vi "Capture@LoadFile__Parameter.vi"(1 "ParamterIn":string) -> (0 "ParamterOut":string)   [LabVIEW 2020]
uses:
  MainFrame/Global.vi
panel:
  out "All Files in Dir":path[](array[path])
  out "Image":T1(plugin-control)
  in  "Picture":string(combo)
  in  "CamName":string(combo)
  in  "Confirm":bool
  # "Capture@General $Capture,$Picture"
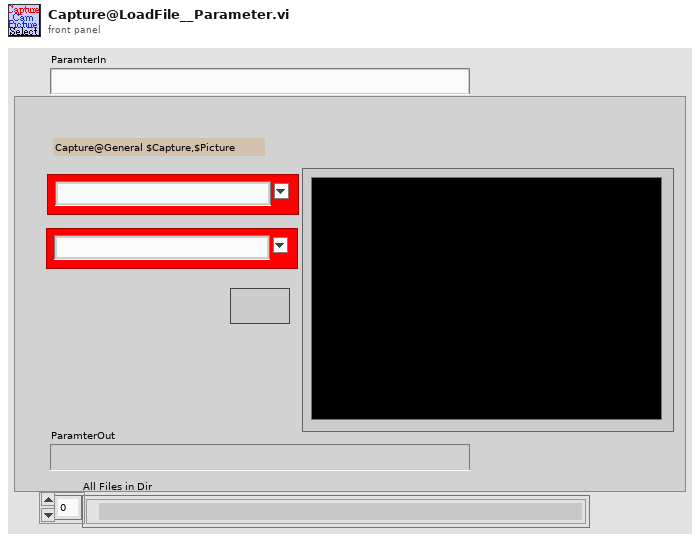
[diagram p1: front panel]
types:
  T1 = typedef "IMAQ Image.ctl" = refnum<image>
  T2 = typedef "Image Type" = u32
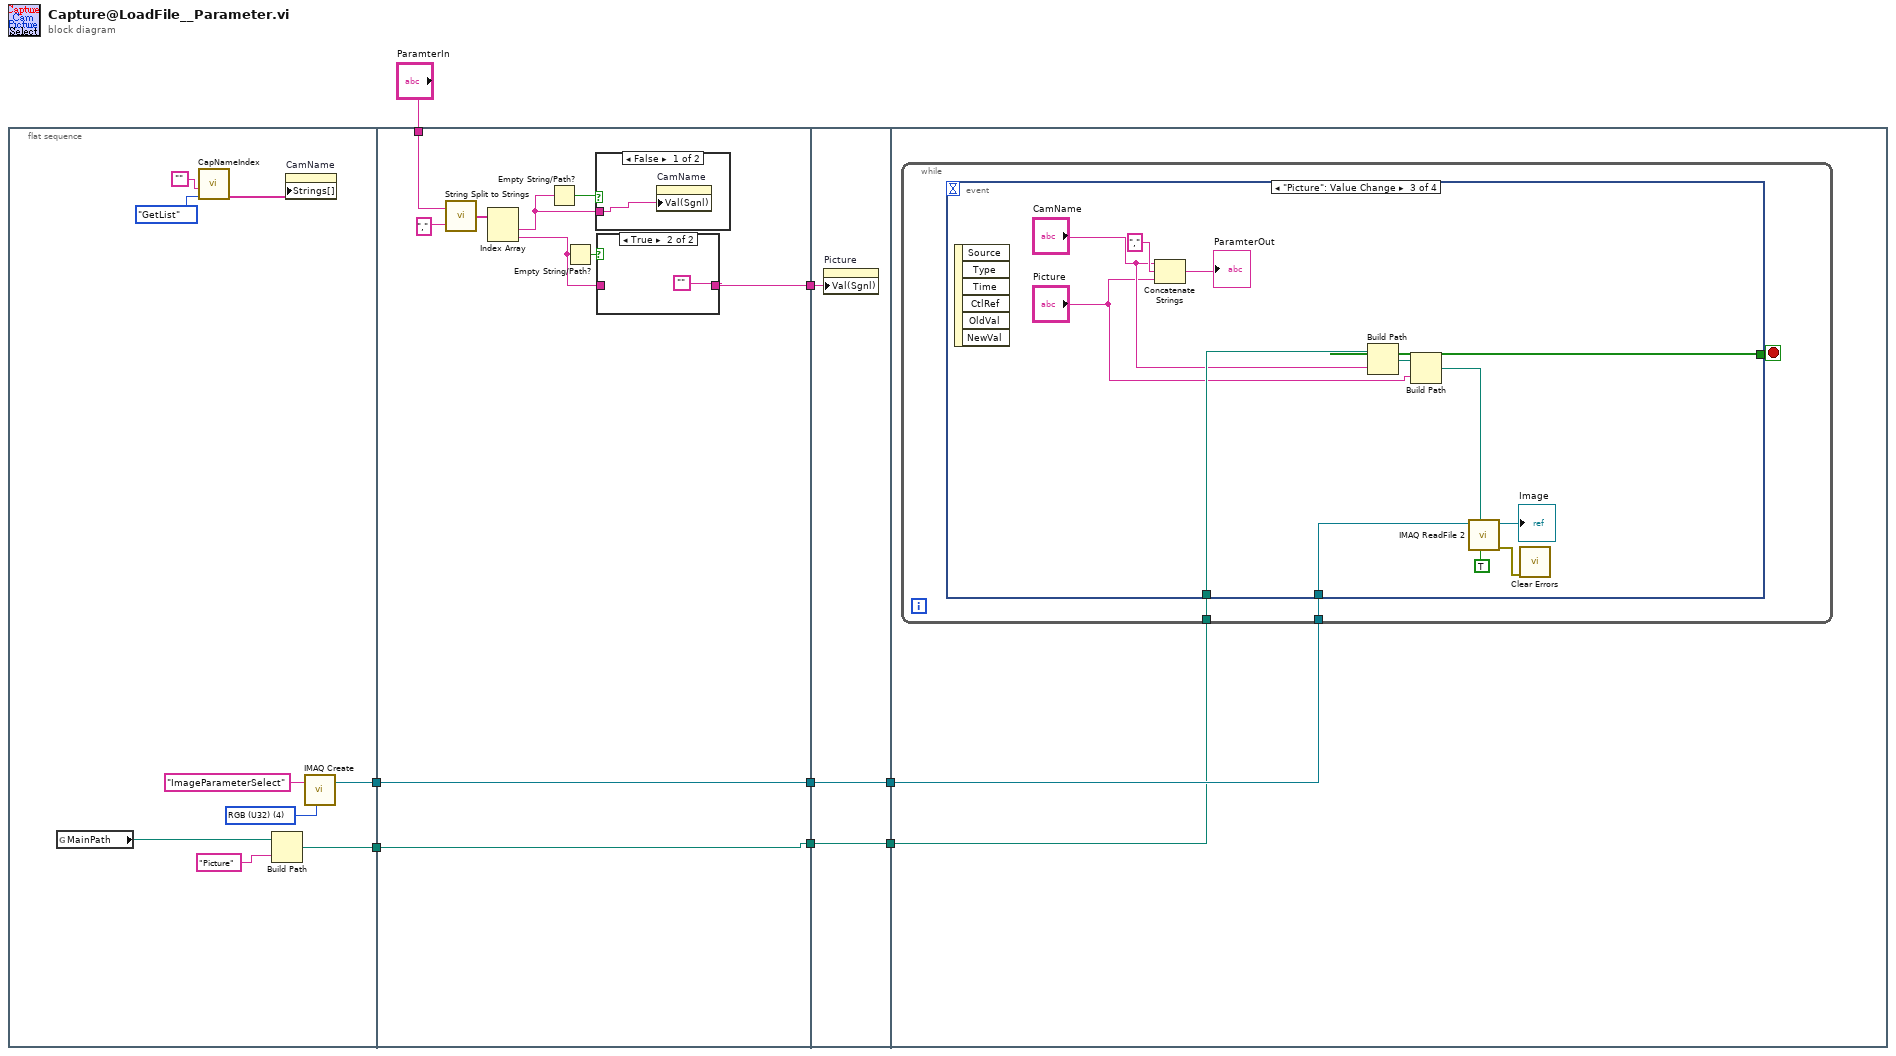
[diagram p0: block diagram]
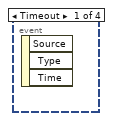
[diagram p4: hidden frame]
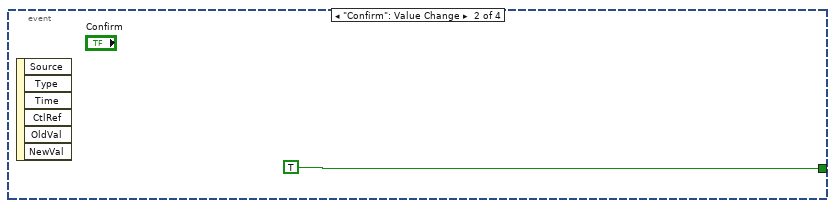
[diagram p5: hidden frame]
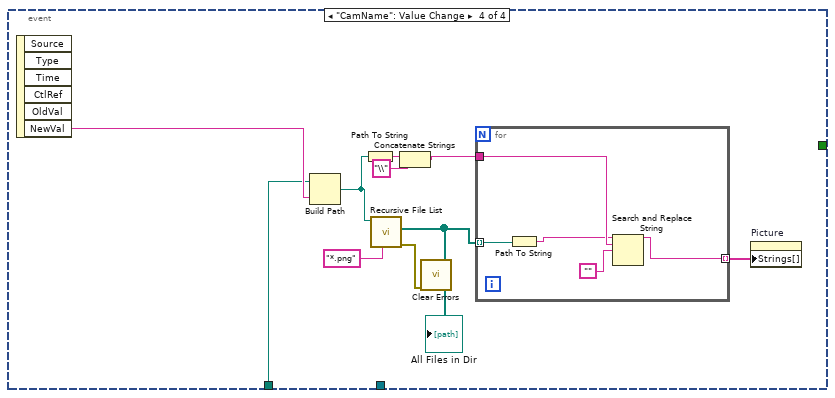
[diagram p6: hidden frame]
diagram:
  n1 = flat-sequence {
    tunnel: [w13] -> w7
    tunnel: [w11] -> w2
    tunnel: "ParamterIn" -> [w25]
    tunnel: w7 -> [w21]
    tunnel: [w21] -> w6
    tunnel: [w19] -> w3
    tunnel: w2 -> [w19]
    tunnel: [w18] -> w1
    tunnel: w6 -> [w33]
    tunnel: [w33] -> w5
    tunnel: [w32] -> w4
    tunnel: w3 -> [w32]
    tunnel: w1 -> [w31]
    tunnel: w5 -> [w35]
    tunnel: w4 -> [w34]
    frame #0 {
      w9 = T2 4 items=["Grayscale (U8)", "Grayscale (I16)", "Grayscale (SGL)", "Complex (CSG)", "RGB (U32)", "HSL (U32)", "RGB (U64)", "Grayscale (U16)"] ("Image Type")
      n2 = global read "Global.vi" "MainPath"() -> (w10:path)
      n3 = call "CapNameIndex.vi"("OP"=enum16{"AddCam", "GetIndex", "Init", "GetList"}."GetList", "CamName"="") -> ("DeviceList"=w16:string[])  [unwired: 2 in, 3 out]
      n4 = Build Path(base path=w10, name or relative path="Picture") -> (appended path=w11:path)
      n5 = property on="CamName" class="CmbBox"("Strings[]"=w16) -> ()  [unwired: 2 in, 2 out]
      n6 = call "IMAQ Create"("Image Name"="ImageParameterSelect", "Image Type"=w9) -> ("New Image"=w13:T1)  [unwired: 3 in, 1 out]
    }
    frame #1 {
      n7 = call "String Split to Strings.vi"("search string/char (-)"=",", "String"=w25) -> ("Array"=w27:string[])
      n8 = Index Array(array=w27) -> (element #1=w20:string, element #2=w22:string)  [unwired: 2 in]
      n9 = Empty String/Path?(string/path=w20) -> (empty?=w24:bool)
      n10 = Empty String/Path?(string/path=w22) -> (empty?=w23:bool)
      n11 = case shown="False" w24 {
        tunnel: w20 -> [w30 _]
        frame False {
          n12 = property on="CamName" class="CmbBox"("Val(Sgnl)"=w30) -> ()  [unwired: 2 in, 2 out]
        }
        frame True {
        }
      }
      n13 = case shown="True" w23 {
        tunnel: [w28 ""] -> w18
        tunnel: w22 -> [w28 _]
        frame False {
        }
        frame True {
        }
      }
    }
    frame #2 {
      n14 = property on="Picture" class="CmbBox"("Val(Sgnl)"=w31) -> ()  [unwired: 2 in, 2 out]
    }
    frame #3 {
      n15 = while {
        tunnel: w35 -> [w37]
        tunnel: w34 -> [w36]
        stop <- w38 stop-if-true
        n16 = event shown="[2] \"Picture\": Value Change" {
          selector: _ -> [_ _ _ _]
          dyn-events: _ -> [_ _ _ _]
          timeout: _ -> [_ _ _ _]
          tunnel: [_ TRUE _ _] -> w38
          tunnel: w37 -> [_ _ w48 _]
          tunnel: w36 -> [_ _ w47 w55]
          event Timeout {
            n17 = event-data() -> ()  [unwired: 1 in, 3 out]
          }
          event "Confirm": Value Change {
            n18 = event-data() -> ()  [unwired: 1 in, 6 out]
          }
          event "Picture": Value Change {
            n19 = event-data() -> ()  [unwired: 1 in, 6 out]
            n20 = Concatenate Strings("CamName", "," ("string"), "Picture") -> (→"ParamterOut":string)
            n21 = Build Path(base path=w47, name or relative path="CamName") -> (appended path=w45:path)
            n22 = Build Path(base path=w45, name or relative path="Picture") -> (appended path=w43:path)
            n23 = call "IMAQ ReadFile 2"("Use File Path Image Type"=TRUE, "File Path"=w43, "Image"=w48) -> ("error out"=w42:errorcluster, "Image Out"=→"Image":T1)  [unwired: 4 in, 3 out]
            n24 = call <vilib>:"Clear Errors.vi"("error in (no error)"=w42) -> ()  [unwired: 5 in, 2 out]
          }
          event "CamName": Value Change {
            n25 = event-data() -> ("NewVal"=w57:string)  [unwired: 1 in, 5 out]
            n26 = Build Path(base path=w55, name or relative path=w57) -> (appended path=w54:path)
            n27 = Path To String(path=w54) -> (string=w53:string)
            n28 = call <vilib>:"Recursive File List.vi"("pattern"="*.png", "Folder Path"=w54) -> ("error out"=w56:errorcluster, "All Files in Dir"=w59:path[])  [unwired: 5 in, 3 out]
            "All Files in Dir" <- w59
            n29 = Concatenate Strings(w53, "\\" ("string")) -> (w51:string)
            n30 = call <vilib>:"Clear Errors.vi"("error in (no error)"=w56) -> ()  [unwired: 5 in, 2 out]
            n31 = for {
              tunnel: w59 -> [w65] mode=indexing
              tunnel: [w61] -> w60 mode=indexing
              tunnel: w51 -> [w63]
              n32 = Path To String(path=w65) -> (string=w62:string)
              n33 = Search and Replace String(input string=w62, search string=w63, replace string="") -> (result string=w61:string)  [unwired: 5 in, 3 out]
            }
            n34 = property on="Picture" class="CmbBox"("Strings[]"=w60) -> ()  [unwired: 2 in, 2 out]
          }
        }
      }
    }
  }
